vi "Evaluate Part 1.vi"() -> ()   [LabVIEW 2020]
panel:
  in  "Input":string
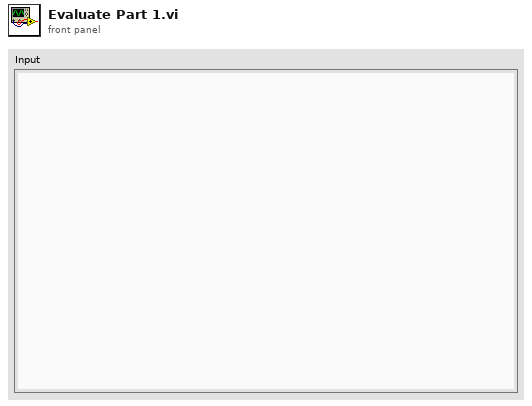
[diagram p1: front panel]
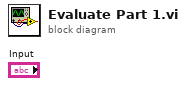
[diagram p0: block diagram]
diagram:
